vi "Image to UTM.vi"(2 "Image Descriptor":T4={"Upper-Left Corner Coordinates"={"UTM Zone"=0.0, "Hemisphere"=enum."North", "East"=0.0, "North"=0.0}, "Meters/Pixel"=42.294203}, 3 "Y":i32, 4 "X":i32) -> (0 "Waypoint":T1, 1 "UTM Location":T3)   [LabVIEW 2011]
doc: "Converts image pixels to Lat/Lon coordinates using an Image Descriptor."
uses:
  0-Image Descriptor.ctl
  2-Think/2 Typedefs/UTM Location.ctl
  0x2-OCU-Think Comm/0x2 Typedefs/ocuWaypoint.ctl
  0x2-OCU-Think Comm/0x2 Typedefs/waypointTypes.ctl
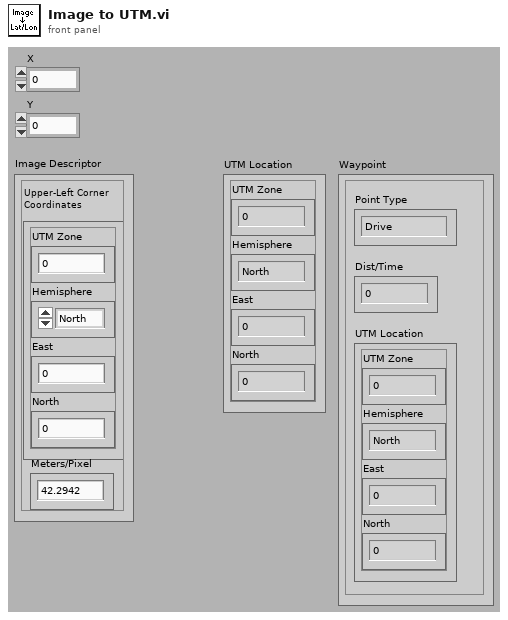
[diagram p1: front panel]
types:
  T1 = typedef "ocuWaypoint.ctl" = cluster{"Point Type":T2, "Dist/Time":dbl, "UTM Location":T3}
  T2 = typedef "waypointTypes.ctl" = enum16{"Drive", "Round Port", "Round Starboard", "Stay"}
  T3 = typedef "UTM Location.ctl" = cluster{"UTM Zone":dbl, "Hemisphere":enum16{"North", "South"}, "East":dbl, "North":dbl}
  T4 = typedef "0-Image Descriptor.ctl" = cluster{"Upper-Left Corner Coordinates":T3, "Meters/Pixel":dbl}
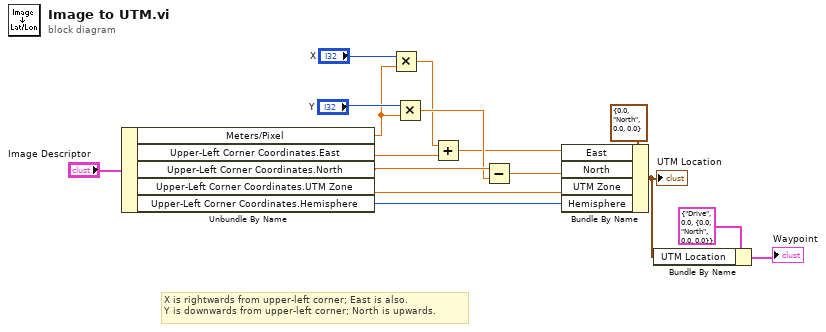
[diagram p0: block diagram]
diagram:
  # "X is rightwards from upper-left corner; East is also.\nY is downwards from upper-left corner; North is upwards."
  n1 = Unbundle By Name("Image Descriptor") -> ("Meters/Pixel"=w10:dbl, "Upper-Left Corner Coordinates.East"=w9:dbl, "Upper-Left Corner Coordinates.North"=w8:dbl, "Upper-Left Corner Coordinates.UTM Zone"=w14:dbl, "Upper-Left Corner Coordinates.Hemisphere"=w13:enum16{"North", "South"})
  n2 = Multiply(x="X", y=w10) -> (x*y=w6:dbl)
  n3 = Multiply(x="Y", y=w10) -> (x*y=w7:dbl)
  n4 = Add(x=w6, y=w9) -> (x+y=w5:dbl)
  n5 = Subtract(x=w8, y=w7) -> (x-y=w4:dbl)
  n6 = Bundle By Name(cluster=T3 {"UTM Zone"=0.0, "Hemisphere"=enum."North", "East"=0.0, "North"=0.0} ("UTM Location 2"), "East"=w5, "North"=w4, "UTM Zone"=w14, "Hemisphere"=w13) -> (w1:T3)
  "UTM Location" <- w1
  n7 = Bundle By Name(cluster=T1 {"Point Type"=enum."Drive", "Dist/Time"=0.0, "UTM Location"={"UTM Zone"=0.0, "Hemisphere"=enum."North", "East"=0.0, "North"=0.0}} ("Waypoint 2"), "UTM Location"=w1) -> (→"Waypoint":T1)
